vi "MenuStrip.vi"(5 "DropDownDirection":i32(ring)=7 items=["AboveLeft"=0, "AboveRight"=1, "BelowLeft"=2, "BelowRight"=3, "Left"=4, "Right"=5, "Default"=7], 6 "LayoutStyle":i32(ring) items=["StackWithOverflow", "HorizontalStackWithOverflow", "VerticalStackWithOverflow", "Flow", "Table"], 7 "TextDirection":i32(ring)=1 items=["Inherit", "Horizontal", "Vertical90", "Vertical270"], 10 "error in (no error)":errorcluster, 11 "MenuStrip":refnum<k24>) -> (2 "error out":errorcluster, 3 "MenuStrip out":refnum<class "MGI_MenuStrip.lvclass">)   [LabVIEW 2016, in "MGI_MenuStrip.lvclass"]
doc: "Creates a .NET MenuStrip. The menu strip input should be a System.Windows.Forms.MenuStrips .NET control on the front panel of your VI.\n\nAuthored by Derek E. Trepanier\nsupport@mooregoodideas.com\nwww.mooregoodideas.com\n\nCopyright (c) 2012, Moore Good Ideas, Inc.\n\nAll rights reserved.\n\nRedistribution and use in source and binary forms, with or without modification, are permitted provided that the following conditions are met:\n\n * Redistributions of source code must retain the above copyright notice, this list of conditions and the following disclaimer.\n * Redistributions in binary form must reproduce the above copyright notice, this list of conditions and the following disclaimer in the documentation and/or other materials provided with the distribution.\n * Neither the name of Moore Good Ideas, Inc. nor the names of its contributors may be used to endorse or promote products derived from this software without specific prior written permission.\n\nTHIS SOFTWARE IS PROVIDED BY THE COPYRIGHT HOLDERS AND CONTRIBUTORS \"AS IS\" AND ANY EXPRESS OR IMPLIED WARRANTIES, INCLUDING, BUT NOT LIMITED TO, THE IMPLIED WARRANTIES OF MERCHANTABILITY AND FITNESS FOR A PARTICULAR PURPOSE ARE DISCLAIMED. IN NO EVENT SHALL THE COPYRIGHT OWNER OR CONTRIBUTORS BE LIABLE FOR ANY DIRECT, INDIRECT, INCIDENTAL, SPECIAL, EXEMPLARY, OR CONSEQUENTIAL DAMAGES (INCLUDING, BUT NOT LIMITED TO, PROCUREMENT OF SUBSTITUTE GOODS OR SERVICES; LOSS OF USE, DATA, OR PROFITS; OR BUSINESS INTERRUPTION) HOWEVER CAUSED AND ON ANY THEORY OF LIABILITY, WHETHER IN CONTRACT, STRICT LIABILITY, OR TORT (INCLUDING NEGLIGENCE OR OTHERWISE) ARISING IN ANY WAY OUT OF THE USE OF THIS SOFTWARE, EVEN IF ADVISED OF THE POSSIBILITY OF SUCH DAMAGE."
uses:
  <userlib>/_MGI/Menu Building/MenuTypes/MenuStrip/MGI_MenuStrip.lvclass
  System.Windows.Forms
  <userlib>/_MGI/Menu Building/MenuTypes/MenuStrip/MGI_MenuStrip.lvclass/MGI_MenuStrip.ctl
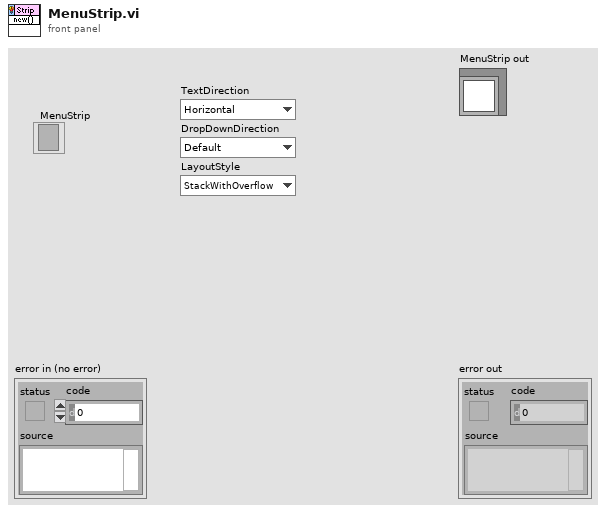
[diagram p1: front panel]
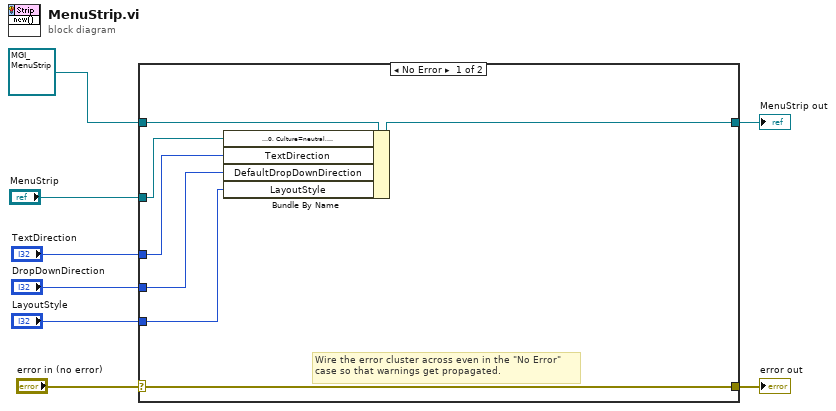
[diagram p0: block diagram]
diagram:
  n1 = case shown="No Error" "error in (no error)" {
    selector: "error in (no error)" -> [w14 w17]
    tunnel: [w14 w17] -> w7
    tunnel: [w13 w16] -> w5
    tunnel: refnum<class "MGI_MenuStrip.lvclass"> refnum ("MenuStrip in") -> [w15 w16]
    tunnel: "MenuStrip" -> [w12 _]
    tunnel: "TextDirection" -> [w11 _]
    tunnel: "DropDownDirection" -> [w10 _]
    tunnel: "LayoutStyle" -> [w9 _]
    frame No Error {
      # "Wire the error cluster across even in the \"No Error\"\ncase so that warnings get propagated."
      n2 = Bundle By Name(cluster=w15, "MenuStrip"=w12, "TextDirection"=w11, "DefaultDropDownDirection"=w10, "LayoutStyle"=w9) -> (w13:refnum<class "MGI_MenuStrip.lvclass">)
    }
    frame Error {
    }
  }
  "error out" <- w7
  "MenuStrip out" <- w5
